vi "Get Daemon Connections.vi"(8 "error in (no error)":errorcluster, 11 "Modbus slave in":refnum<class "Modbus Slave.lvclass">) -> (0 "error out":errorcluster, 2 "connections":T1(array[cluster]), 3 "Modbus slave out":refnum<class "Modbus Slave.lvclass">)   [LabVIEW 2020, in "Modbus Slave.lvclass"]
doc: "<B>TCP Connection List</B> returns the information about the TCP connections established to the Modbus slave. This information shows you the IP address and connection error of a Modbus master and whether this Modbus master is connected to the Modbus slave. To get this property, ensure that you wire a TCP Modbus slave to the <B>reference</B> input. Otherwise, LabVIEW returns error code -389106."
uses:
  <vilib>/Modbus/slave/Modbus Slave.lvclass
  <vilib>/Modbus/slave/Modbus Slave.lvclass/Modbus Slave.ctl
  <vilib>/Modbus/subvis/Protocol/TCP/TCP Slave/TCP Slave.lvclass
  <vilib>/Modbus/subvis/Protocol/TCP/TCP Slave/TCP Slave.lvclass/TCP Slave.ctl
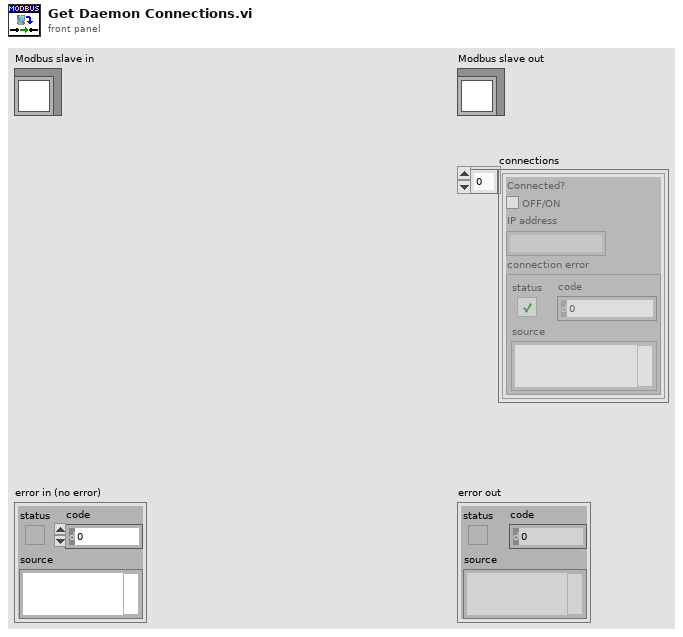
[diagram p1: front panel]
types:
  T1 = cluster{"Connected?":bool, "IP address":string, "connection error":errorcluster}[]
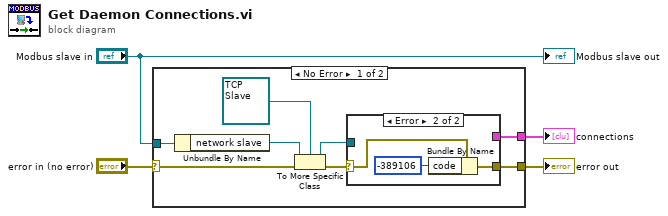
[diagram p0: block diagram]
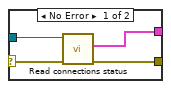
[diagram p2: hidden frame]
diagram:
  n1 = case shown="No Error" "error in (no error)" {
    selector: "error in (no error)" -> [w12 w20]
    tunnel: [w9 _] -> w2
    tunnel: [w8 w20] -> w3
    tunnel: "Modbus slave in" -> [w7 _]
    frame No Error {
      n2 = Unbundle By Name(w7) -> ("network slave"=w6:refnum<class "Network Slave.lvclass">)
      n3 = To More Specific Class(target class=refnum<class "TCP Slave.lvclass"> refnum ("TCP Slave"), reference=w6, error in=w12) -> (specific class reference=w10:refnum<class "TCP Slave.lvclass">, error out=w11:errorcluster)
      n4 = case shown="Error" w11 {
        selector: w11 -> [w15 w19]
        tunnel: w10 -> [w16 _]
        tunnel: [w13 _] -> w9
        tunnel: [w14 w18] -> w8
        frame No Error {
          n5 = call <vilib>:"Read connections status.vi"("error in (no error)"=w15, "TCP slave in"=w16) -> ("error out"=w14:errorcluster, "connections"=w13:T1)  [unwired: 7 in, 1 out]
        }
        frame Error {
          n6 = Bundle By Name(cluster=w19, "code"=-389106) -> (w18:errorcluster)
        }
      }
    }
    frame Error {
    }
  }
  "error out" <- w3
  "connections" <- w2
  "Modbus slave out" <- "Modbus slave in"
